vi "Teleop.vi"(10 "Match Info":T1={"Autonomous Elapsed Seconds"=0.0, "TeleOp Elapsed Seconds"=0.0, "Disabled Elapsed Seconds"=0.0, "Visited Autonomous"=FALSE, "Visited TeleOp"=FALSE, "Visited Disabled"=FALSE, "Autonomous Settings"={"Autonomous Style"=enum."Independent", "VI Refnum"=refnum}}, 11 "Call Context":T2) -> ()   [LabVIEW 2019]
doc: "This VI is called for each enabled TeleOp packet received from the DS. It is typically used to read from joysticks and other inputs and update I/O or setpoints for timed control loops. It should complete and return within 20 milliseconds or risk missing DS packets."
uses:
  <vilib>/Rock Robotics/WPI/DriverStation/WPI_DriverStationDerivedRobotMode.ctl
  <vilib>/Rock Robotics/WPI/DriverStation/WPI_DriverStationMatch Info.ctl
  Framework/Robot Global Data.vi
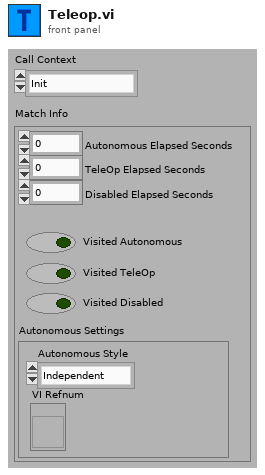
[diagram p1: front panel]
types:
  T1 = typedef "WPI_DriverStationMatch Info.ctl" = cluster{"Autonomous Elapsed Seconds":dbl, "TeleOp Elapsed Seconds":dbl, "Disabled Elapsed Seconds":dbl, "Visited Autonomous":bool, "Visited TeleOp":bool, "Visited Disabled":bool, "Autonomous Settings":cluster{"Autonomous Style":enum16{"Iterative", "Independent"}, "VI Refnum":refnum<vi>}}
  T2 = typedef "WPI_DriverStationDerivedRobotMode.ctl" = enum16{"Init", "Execute", "Stop"}
  T3 = typedef "Command Status Info.ctl" = cluster{"Name":string, "Status":T4, "notifier out":T5}
  T4 = typedef "Completion Status.ctl" = enum16{"Successful", "Aborted", "Incomplete"}
  T5 = typedef "Completion Notifier.ctl" = refnum<notifier>
  T6 = cluster{"XAngle":dbl, "YAngle":dbl, "ZAngle":dbl}
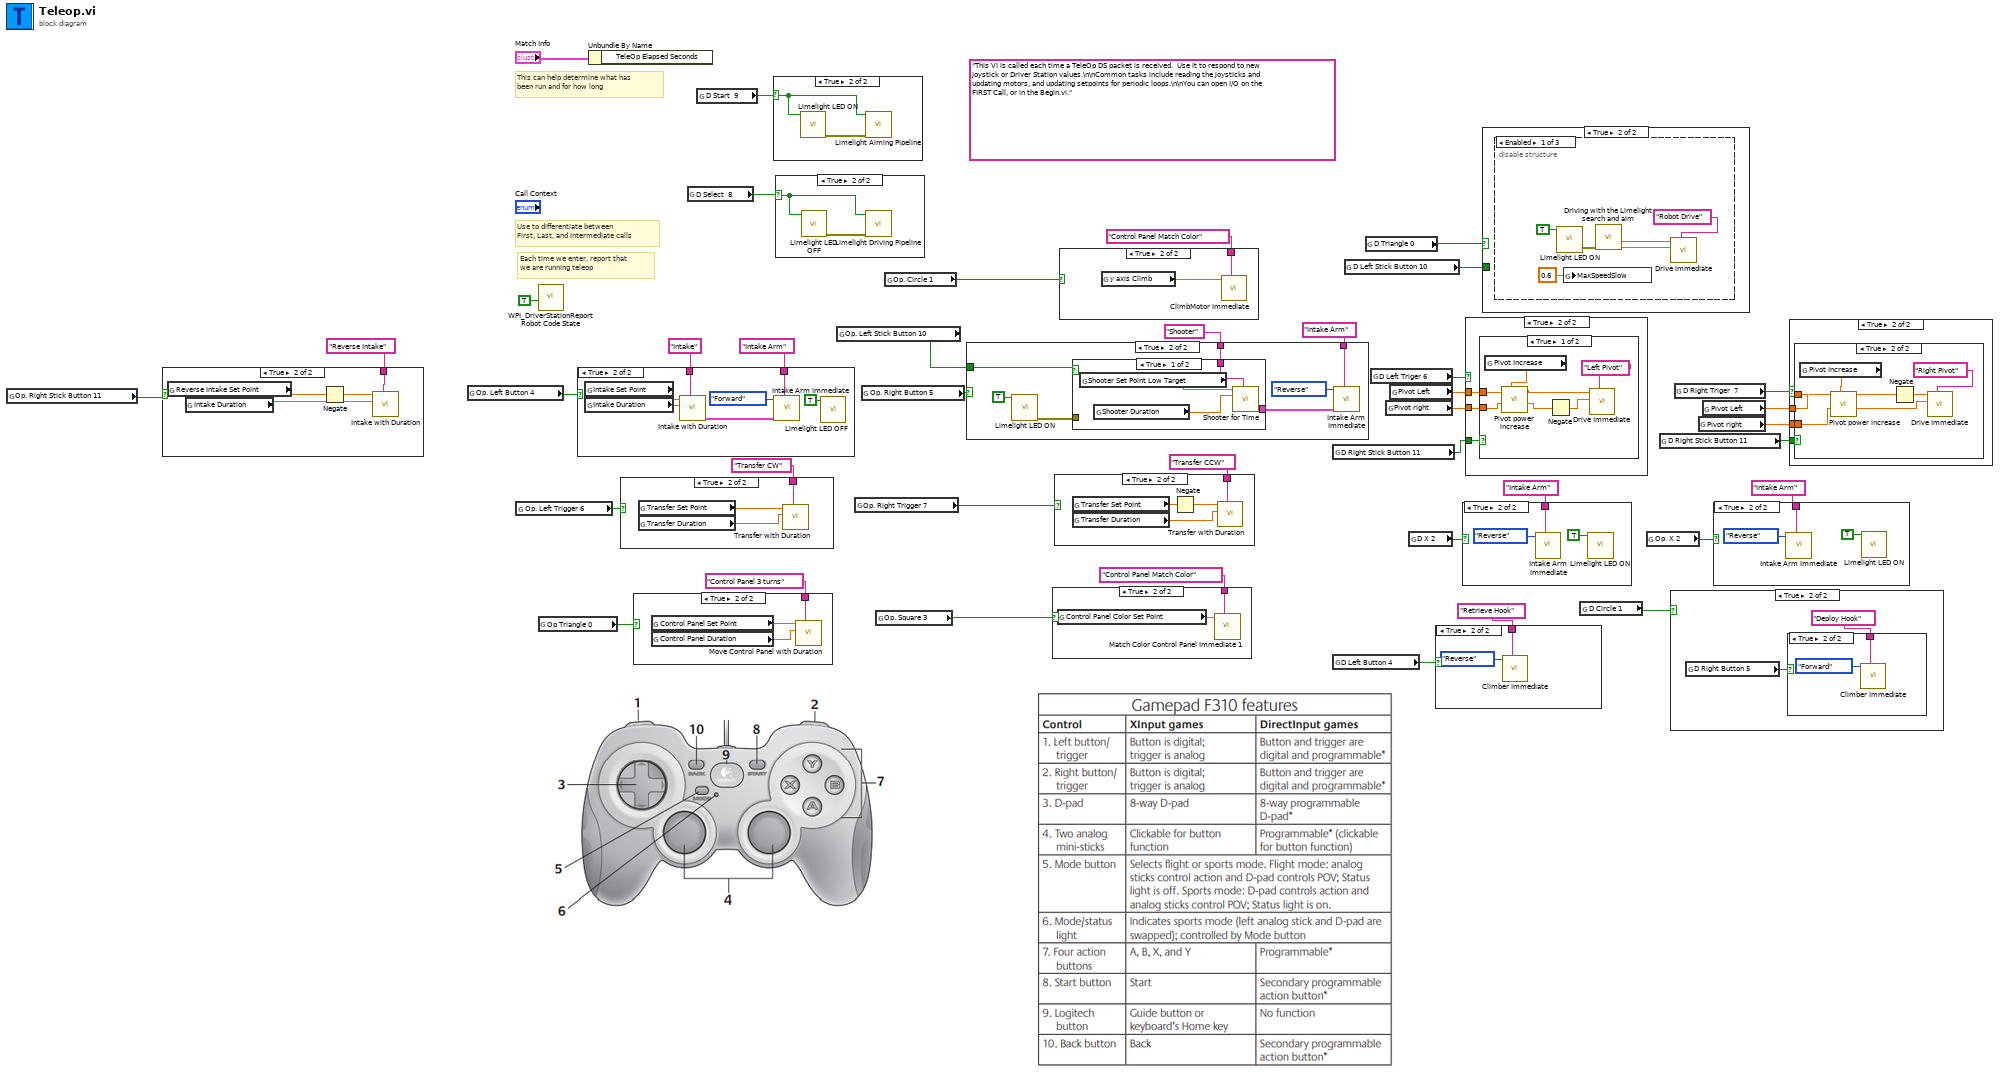
[diagram p0: block diagram]
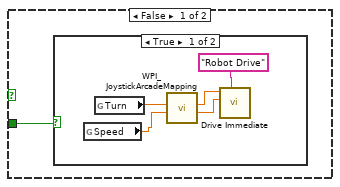
[diagram p10: hidden frame]
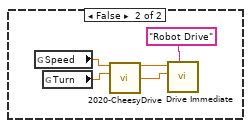
[diagram p11: hidden frame]
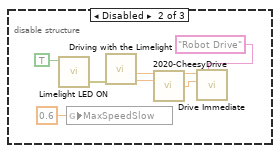
[diagram p12: hidden frame]
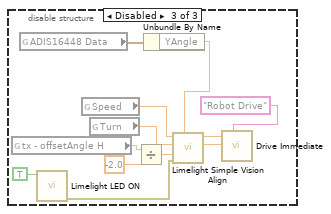
[diagram p13: hidden frame]
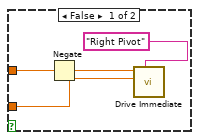
[diagram p18: hidden frame]
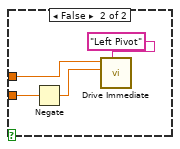
[diagram p20: hidden frame]
diagram:
  (unwired) "This VI is called each time a TeleOp DS packet is received.  Use it to respond to new joystick or Driver Station values.\n\nCommon tasks include reading the joysticks and updating motors, and updating setpoints for periodic loops.\n\nYou can open I/O on the FIRST Call, or in the Begin.vi."
  # "Each time we enter, report that\nwe are running teleop"
  # "Use to differentiate between\nFirst, Last, and Intermediate calls"
  # "This can help determine what has\nbeen run and for how long"
  n1 = global read "Robot Global Data.vi" "Op. Right Stick Button 11"() -> (w3:bool)
  n2 = case shown="True" w3 {
    tunnel: "Reverse Intake" ("refnum name") -> [_ w44]
    frame False {
    }
    frame True {
      n3 = global read "Robot Global Data.vi" "Reverse Intake Set Point"() -> (w43:dbl)
      n4 = global read "Robot Global Data.vi" "Intake Duration"() -> (w42:dbl)
      n5 = Negate(x=w43) -> (-x=w41:dbl)
      n6 = call "Intake with Duration.vi"("Description"=w44, "Duration (s)"=w42, "Setpoint"=w41) -> ()  [unwired: 8 in, 1 out]
    }
  }
  n7 = global read "Robot Global Data.vi" "Op. Left Button 4"() -> (w38:bool)
  n8 = global read "Robot Global Data.vi" "Op. Left Trigger 6"() -> (w32:bool)
  n9 = call <vilib>:"WPI_DriverStationReport Robot Code State.vi"("TeleOp"=TRUE ("Autonomous")) -> ()  [unwired: 10 in, 1 out]
  n10 = global read "Robot Global Data.vi" "Op Triangle 0"() -> (w25:bool)
  n11 = case shown="True" w38 {
    tunnel: "Intake" ("refnum name") -> [_ w51]
    tunnel: "Intake Arm" ("refnum name") -> [_ w47]
    frame False {
    }
    frame True {
      n12 = global read "Robot Global Data.vi" "Intake Set Point"() -> (w50:dbl)
      n13 = global read "Robot Global Data.vi" "Intake Duration"() -> (w49:dbl)
      n14 = call "Intake with Duration.vi"("Description"=w51, "Duration (s)"=w49, "Setpoint"=w50) -> ("Command Info Out"=w46:T3)  [unwired: 8 in]
      n15 = call "Intake Arm Immediate.vi"("Description"=w47, "Command Info In"=w46, "Relay Value"=enum16{"Off", "On", "Forward", "Reverse"}."Forward") -> ()  [unwired: 8 in, 1 out]
      n16 = call "Limelight LED OFF.vi"("D Select  8"=TRUE) -> ()  [unwired: 10 in, 1 out]
    }
  }
  n17 = Unbundle By Name("Match Info") -> ()  [unwired: 1 out]
  n18 = case shown="True" w32 {
    tunnel: "Transfer CW" ("refnum name") -> [_ w54]
    frame False {
    }
    frame True {
      n19 = global read "Robot Global Data.vi" "Transfer Set Point"() -> (w53:dbl)
      n20 = global read "Robot Global Data.vi" "Transfer Duration"() -> (w52:dbl)
      n21 = call "Transfer with Duration.vi"("Description"=w54, "Duration (s)"=w52, "Setpoint"=w53) -> ()  [unwired: 8 in, 1 out]
    }
  }
  n22 = case shown="True" w25 {
    tunnel: "Control Panel 3 turns" ("refnum name") -> [_ w57]
    frame False {
    }
    frame True {
      n23 = global read "Robot Global Data.vi" "Control Panel Set Point"() -> (w56:dbl)
      n24 = global read "Robot Global Data.vi" "Control Panel Duration"() -> (w55:dbl)
      n25 = call "Move Control Panel with Duration.vi"("Description"=w57, "Duration (s)"=w55, "Setpoint"=w56) -> ()  [unwired: 8 in, 1 out]
    }
  }
  n26 = global read "Robot Global Data.vi" "D Select  8"() -> (w1:bool)
  n27 = global read "Robot Global Data.vi" "D Start  9"() -> (w2:bool)
  n28 = case shown="True" w2 {
    selector: w2 -> [_ w58]
    frame False {
    }
    frame True {
      n29 = call "Limelight LED ON.vi"("D Start  9"=w58) -> ("error out"=w59:errorcluster)  [unwired: 10 in]
      n30 = call "Limelight Aiming Pipeline.vi"("error in (no error)"=w59, "Set Pipeline"=w58) -> ()  [unwired: 9 in, 1 out]
    }
  }
  n31 = case shown="True" w1 {
    selector: w1 -> [_ w60]
    frame False {
    }
    frame True {
      n32 = call "Limelight LED OFF.vi"("D Select  8"=w60) -> ("error out"=w61:errorcluster)  [unwired: 10 in]
      n33 = call "Limelight Driving Pipeline.vi"("error in (no error)"=w61, "Set Pipeline"=w60) -> ()  [unwired: 9 in, 1 out]
    }
  }
  n34 = global read "Robot Global Data.vi" "Op. Left Stick Button 10"() -> (w8:bool)
  n35 = global read "Robot Global Data.vi" "Op. Right Trigger 7"() -> (w33:bool)
  n36 = global read "Robot Global Data.vi" "Op. Right Button 5"() -> (w34:bool)
  n37 = global read "Robot Global Data.vi" "Op. Square 3"() -> (w22:bool)
  n38 = global read "Robot Global Data.vi" "Op. Circle 1"() -> (w10:bool)
  n39 = case shown="True" w34 {
    tunnel: "Shooter" ("refnum name") -> [_ w68]
    tunnel: "Intake Arm" ("refnum name") -> [_ w66]
    tunnel: w8 -> [_ w64]
    frame False {
    }
    frame True {
      n40 = call "Limelight LED ON.vi"("D Start  9"=TRUE) -> ("error out"=w62:errorcluster)  [unwired: 10 in]
      n41 = case shown="True" w64 {
        tunnel: w68 -> [w72 w76]
        tunnel: [w69 w73] -> w65
        tunnel: w62 -> [_ _]
        frame True {
          n42 = global read "Robot Global Data.vi" "Shooter Set Point Low Target"() -> (w71:dbl)
          n43 = global read "Robot Global Data.vi" "Shooter Duration"() -> (w70:dbl)
          n44 = call "Shooter for Time.vi"("Description"=w72, "Duration (s)"=w70, "Setpoint"=w71) -> ("Command Info Out"=w69:T3)  [unwired: 8 in]
        }
        frame False {
          n45 = global read "Robot Global Data.vi" "Shooter Set Point"() -> (w75:dbl)
          n46 = global read "Robot Global Data.vi" "Shooter Duration"() -> (w74:dbl)
          n47 = call "Shooter for Time.vi"("Description"=w76, "Duration (s)"=w74, "Setpoint"=w75) -> ("Command Info Out"=w73:T3)  [unwired: 8 in]
        }
      }
      n48 = call "Intake Arm Immediate.vi"("Description"=w66, "Command Info In"=w65, "Relay Value"=enum16{"Off", "On", "Forward", "Reverse"}."Reverse") -> ()  [unwired: 8 in, 1 out]
    }
  }
  n49 = case shown="True" w22 {
    tunnel: "Control Panel Match Color" ("refnum name") -> [_ w78]
    frame False {
    }
    frame True {
      n50 = global read "Robot Global Data.vi" "Control Panel Color Set Point"() -> (w77:dbl)
      n51 = call "Match Color Control Panel Immediate 1.vi"("Description"=w78, "Setpoint"=w77) -> ()  [unwired: 9 in, 1 out]
    }
  }
  n52 = case shown="True" w33 {
    tunnel: "Transfer CCW" ("refnum name") -> [_ w82]
    frame False {
    }
    frame True {
      n53 = global read "Robot Global Data.vi" "Transfer Set Point"() -> (w80:dbl)
      n54 = global read "Robot Global Data.vi" "Transfer Duration"() -> (w79:dbl)
      n55 = Negate(x=w80) -> (-x=w81:dbl)
      n56 = call "Transfer with Duration.vi"("Description"=w82, "Duration (s)"=w79, "Setpoint"=w81) -> ()  [unwired: 8 in, 1 out]
    }
  }
  n57 = case shown="True" w10 {
    tunnel: "Control Panel Match Color" ("refnum name") -> [_ w84]
    frame False {
    }
    frame True {
      n58 = global read "Robot Global Data.vi" "y axis Climb"() -> (w83:dbl)
      n59 = call "ClimbMotor Immediate.vi"("Description"=w84, "Setpoint"=w83) -> ()  [unwired: 9 in, 1 out]
    }
  }
  n60 = global read "Robot Global Data.vi" "D Right Stick Button 11"() -> (w5:bool)
  n61 = global read "Robot Global Data.vi" "D Left Button 4"() -> (w15:bool)
  n62 = global read "Robot Global Data.vi" "D Left Stick Button 10"() -> (w7:bool)
  n63 = global read "Robot Global Data.vi" "D Triangle 0"() -> (w16:bool)
  n64 = global read "Robot Global Data.vi" "D Left Triger 6"() -> (w30:bool)
  n65 = global read "Robot Global Data.vi" "Pivot right"() -> (w19:dbl)
  n66 = global read "Robot Global Data.vi" "Pivot Left"() -> (w20:dbl)
  n67 = global read "Robot Global Data.vi" "D X 2"() -> (w23:bool)
  n68 = case shown="True" w15 {
    tunnel: "Retrieve Hook" ("refnum name") -> [_ w85]
    frame False {
    }
    frame True {
      n69 = call "Climber Immediate.vi"("Description"=w85, "Value"=enum16{"Off", "On", "Forward", "Reverse"}."Reverse" ("Relay Value")) -> ()  [unwired: 9 in, 1 out]
    }
  }
  n70 = case shown="True" w23 {
    tunnel: "Intake Arm" ("refnum name") -> [_ w88]
    frame False {
    }
    frame True {
      n71 = call "Intake Arm Immediate.vi"("Description"=w88, "Relay Value"=enum16{"Off", "On", "Forward", "Reverse"}."Reverse") -> ()  [unwired: 9 in, 1 out]
      n72 = call "Limelight LED ON.vi"("D Start  9"=TRUE) -> ()  [unwired: 10 in, 1 out]
    }
  }
  n73 = case shown="True" w30 {
    tunnel: w20 -> [_ w92]
    tunnel: w19 -> [_ w91]
    tunnel: w5 -> [_ w90]
    frame False {
    }
    frame True {
      n74 = case shown="True" w90 {
        tunnel: w92 -> [w97 w102]
        tunnel: w91 -> [w96 w101]
        frame True {
          n75 = global read "Robot Global Data.vi" "Pivot Increase"() -> (w93:dbl)
          n76 = call "Pivot power increase.vi"("Pivot Increase"=w93, "Input Pivot Right"=w96, "Input Pivot Left"=w97) -> ("Output Pivot Right"=w94:dbl, "Output Pivot Left"=w95:dbl)  [unwired: 7 in]
          n77 = Negate(x=w94) -> (-x=w98:dbl)
          n78 = call "Drive Immediate.vi"("Description"="Left Pivot", "Right Setpoint"=w98, "Left Setpoint"=w95) -> ()  [unwired: 8 in, 1 out]
        }
        frame False {
          n79 = Negate(x=w101) -> (-x=w100:dbl)
          n80 = call "Drive Immediate.vi"("Description"="Left Pivot", "Right Setpoint"=w100, "Left Setpoint"=w102) -> ()  [unwired: 8 in, 1 out]
        }
      }
    }
  }
  n81 = case shown="True" w16 {
    tunnel: w7 -> [w104 _]
    frame False {
      n82 = case shown="True" w104 {
        frame True {
          n83 = global read "Robot Global Data.vi" "Speed"() -> (w107:dbl)
          n84 = global read "Robot Global Data.vi" "Turn"() -> (w108:dbl)
          n85 = call <vilib>:"WPI_JoystickArcadeMapping.vi"("Y axis value"=w107, "X axis value"=w108) -> ("Right Motor Value"=w105:dbl, "Left Motor Value"=w106:dbl)  [unwired: 8 in]
          n86 = call "Drive Immediate.vi"("Description"="Robot Drive", "Right Setpoint"=w105, "Left Setpoint"=w106) -> ()  [unwired: 8 in, 1 out]
        }
        frame False {
          n87 = global read "Robot Global Data.vi" "Speed"() -> (w111:dbl)
          n88 = global read "Robot Global Data.vi" "Turn"() -> (w112:dbl)
          n89 = call "2020-CheesyDrive.vi"("Throttle"=w111, "Wheel"=w112) -> ("Left PWM"=w113:dbl, "Right PWM"=w114:dbl)  [unwired: 12 in]
          n90 = call "Drive Immediate.vi"("Description"="Robot Drive", "Right Setpoint"=w114, "Left Setpoint"=w113) -> ()  [unwired: 8 in, 1 out]
        }
      }
    }
    frame True {
      n91 = disable-structure shown="Enabled" {
        frame Enabled {
          n92 = call "Limelight LED ON.vi"("D Start  9"=TRUE) -> ("error out"=w119:errorcluster)  [unwired: 10 in]
          n93 = global write "Robot Global Data.vi" "MaxSpeedSlow"(0.6 ("MaxSpeedSlow")) -> ()
          n94 = call "Driving with the Limelight search and aim.vi"("error in (no error)"=w119) -> ("TurnCommand"=w115:dbl, "SpeedCommand"=w116:dbl)  [unwired: 8 in, 1 out]
          n95 = call "Drive Immediate.vi"("Description"="Robot Drive", "Right Setpoint"=w115, "Left Setpoint"=w116) -> ()  [unwired: 8 in, 1 out]
        }
        frame Disabled {
          n96 = call "Limelight LED ON.vi"("D Start  9"=TRUE) -> ("error out"=w123:errorcluster)  [unwired: 10 in]
          n97 = global write "Robot Global Data.vi" "MaxSpeedSlow"(0.6 ("MaxSpeedSlow")) -> ()
          n98 = call "Driving with the Limelight.vi"("error in (no error)"=w123) -> ("TurnCommand"=w124:dbl, "SpeedCommand"=w125:dbl)  [unwired: 8 in, 1 out]
          n99 = call "2020-CheesyDrive.vi"("Throttle"=w125, "Wheel"=w124) -> ("Left PWM"=w127:dbl, "Right PWM"=w128:dbl)  [unwired: 12 in]
          n100 = call "Drive Immediate.vi"("Description"="Robot Drive", "Right Setpoint"=w128, "Left Setpoint"=w127) -> ()  [unwired: 8 in, 1 out]
        }
        frame Disabled {
          n101 = global read "Robot Global Data.vi" "tx - offsetAngle H"() -> (w134:dbl)
          n102 = global read "Robot Global Data.vi" "ADIS16448 Data"() -> (w130:T6)
          n103 = call "Limelight LED ON.vi"("D Start  9"=TRUE) -> ("error out"=w138:errorcluster)  [unwired: 10 in]
          n104 = global read "Robot Global Data.vi" "Speed"() -> (w132:dbl)
          n105 = global read "Robot Global Data.vi" "Turn"() -> (w131:dbl)
          n106 = Divide(x=w134, y=-2.0) -> (x/y=w135:dbl)
          n107 = Unbundle By Name(w130) -> ("YAngle"=w129:dbl)
          n108 = call "Limelight Simple Vision Align.vi"("Gyro Angle"=w129, "error in (no error)"=w138, "Target Offset"=w135, "Manual Turn"=w131, "Throttle"=w132) -> ("Right Power"=w136:dbl, "Left Power"=w137:dbl)  [unwired: 5 in]
          n109 = call "Drive Immediate.vi"("Description"="Robot Drive", "Right Setpoint"=w136, "Left Setpoint"=w137) -> ()  [unwired: 8 in, 1 out]
        }
      }
    }
  }
  n110 = global read "Robot Global Data.vi" "D Circle 1"() -> (w9:bool)
  n111 = global read "Robot Global Data.vi" "Op. X 2"() -> (w13:bool)
  n112 = global read "Robot Global Data.vi" "D Right Stick Button 11"() -> (w6:bool)
  n113 = case shown="True" w9 {
    frame False {
    }
    frame True {
      n114 = global read "Robot Global Data.vi" "D Right Button 5"() -> (w141:bool)
      n115 = case shown="True" w141 {
        tunnel: "Deploy Hook" ("refnum name") -> [_ w143]
        frame False {
        }
        frame True {
          n116 = call "Climber Immediate.vi"("Description"=w143, "Value"=enum16{"Off", "On", "Forward", "Reverse"}."Forward" ("Relay Value")) -> ()  [unwired: 9 in, 1 out]
        }
      }
    }
  }
  n117 = global read "Robot Global Data.vi" "D Right Triger  7"() -> (w29:bool)
  n118 = global read "Robot Global Data.vi" "Pivot right"() -> (w17:dbl)
  n119 = global read "Robot Global Data.vi" "Pivot Left"() -> (w18:dbl)
  n120 = case shown="True" w13 {
    tunnel: "Intake Arm" ("refnum name") -> [_ w146]
    frame False {
    }
    frame True {
      n121 = call "Intake Arm Immediate.vi"("Description"=w146, "Relay Value"=enum16{"Off", "On", "Forward", "Reverse"}."Reverse") -> ()  [unwired: 9 in, 1 out]
      n122 = call "Limelight LED ON.vi"("D Start  9"=TRUE) -> ()  [unwired: 10 in, 1 out]
    }
  }
  n123 = case shown="True" w29 {
    tunnel: w18 -> [_ w150]
    tunnel: w17 -> [_ w149]
    tunnel: w6 -> [_ w148]
    frame False {
    }
    frame True {
      n124 = case shown="True" w148 {
        tunnel: w150 -> [w153 w159]
        tunnel: w149 -> [w152 w158]
        frame False {
          n125 = Negate(x=w153) -> (-x=w151:dbl)
          n126 = call "Drive Immediate.vi"("Description"="Right Pivot", "Right Setpoint"=w152, "Left Setpoint"=w151) -> ()  [unwired: 8 in, 1 out]
        }
        frame True {
          n127 = global read "Robot Global Data.vi" "Pivot Increase"() -> (w155:dbl)
          n128 = call "Pivot power increase.vi"("Pivot Increase"=w155, "Input Pivot Right"=w158, "Input Pivot Left"=w159) -> ("Output Pivot Right"=w156:dbl, "Output Pivot Left"=w157:dbl)  [unwired: 7 in]
          n129 = Negate(x=w157) -> (-x=w160:dbl)
          n130 = call "Drive Immediate.vi"("Description"="Right Pivot", "Right Setpoint"=w156, "Left Setpoint"=w160) -> ()  [unwired: 8 in, 1 out]
        }
      }
    }
  }
